vi "Read ClockParameter.vi"(8 "error in (no error)":errorcluster, 11 "BME_DG_Base in":refnum<class "BME_DG_Base.lvclass">) -> (0 "error out":errorcluster, 1 "PrescalerCrystalOsc":u32, 2 "ClockEnable":bool, 3 "BME_DG_Base out":refnum<class "BME_DG_Base.lvclass">, 4 "ClockSource":T1=1 items=["Internal Oscillator"=1, "External Trigger"=2, "Trigger-> Oscillator"=3, "MasterSlave Bus"=4])   [LabVIEW 2009, in "POLARIS BME DG.lvlib" / "BME_DG_Base.lvclass"]
uses:
  BME_DG_Base.lvclass
  LV-BME Interface/ClockSource.ctl
  BME_DG_Base.lvclass/BME_DG_Base.ctl
  POLARIS BME DG.lvlib
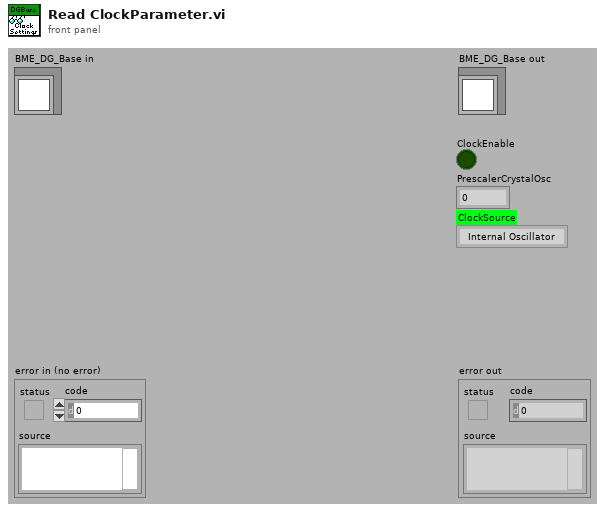
[diagram p1: front panel]
types:
  T1 = typedef "POLARIS BME DG.lvlib/ClockSource.ctl" = i32
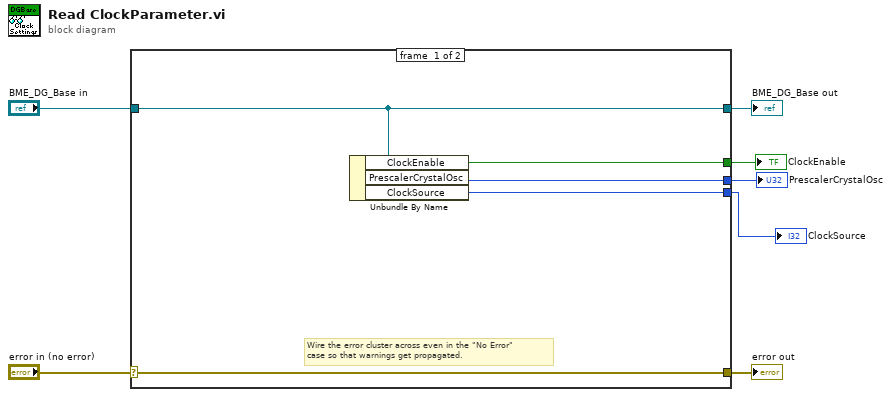
[diagram p0: block diagram]
diagram:
  n1 = case shown="No Error" "error in (no error)" {
    selector: "error in (no error)" -> [w12 w14]
    tunnel: [w12 w14] -> w6
    tunnel: [w11 w13] -> w4
    tunnel: "BME_DG_Base in" -> [w11 w13]
    tunnel: [w10 _] -> w3
    tunnel: [w9 _] -> w2
    tunnel: [w8 _] -> w1
    frame #0 {
      # "Wire the error cluster across even in the \"No Error\"\ncase so that warnings get propagated."
      n2 = Unbundle By Name(w11) -> ("ClockEnable"=w10:bool, "PrescalerCrystalOsc"=w8:u32, "ClockSource"=w9:T1)
    }
    frame #1 {
    }
  }
  "error out" <- w6
  "BME_DG_Base out" <- w4
  "ClockEnable" <- w3
  "PrescalerCrystalOsc" <- w1
  "ClockSource" <- w2
